vi "Write to Hardware.vi"(8 "error in (no error)":errorcluster, 10 "Values in":dbl[](array[numeric]), 11 "NI-XNET CAN Reader Execution Unit in":refnum<class "NI-XNET CAN Reader Execution Unit.lvclass">) -> (0 "error out":errorcluster, 2 "Values out":dbl[](array[numeric]), 3 "NI-XNET CAN Reader Execution Unit out":refnum<class "NI-XNET CAN Reader Execution Unit.lvclass">)   [LabVIEW 2020, in "Communication Bus Template Engine.lvlib" / "Implementation.lvlib" / "NI-XNET CAN Reader Execution Unit.lvclass"]
uses:
  NI-XNET CAN Reader Execution Unit.lvclass
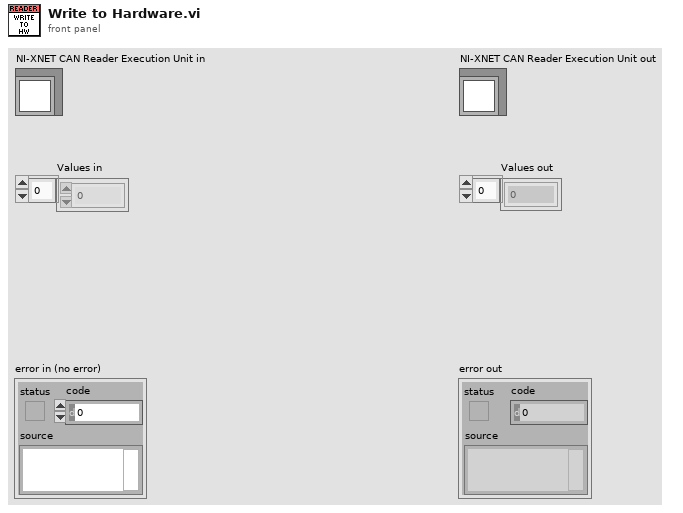
[diagram p1: front panel]
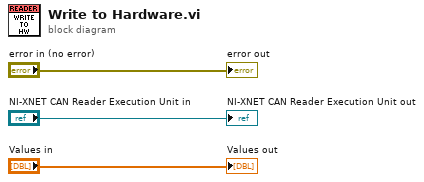
[diagram p0: block diagram]
diagram:
  "error out" <- "error in (no error)"
  "NI-XNET CAN Reader Execution Unit out" <- "NI-XNET CAN Reader Execution Unit in"
  "Values out" <- "Values in"
